vi "ItemByIndex.vi"(7 "LabVIEW Object Type":refnum<class>, 8 "error in (no error)":errorcluster, 10 "Index":i32, 11 "Collection in":refnum<class "CollectionByValue.lvclass">) -> (0 "error out":errorcluster, 1 "found?":bool, 2 "LabVIEW Object":refnum<class>, 3 "Collection out":refnum<class "CollectionByValue.lvclass">)   [LabVIEW 2021, in "Collection.lvlib" / "CollectionByValue.lvclass"]
uses:
  CollectionByValue.lvclass
  CollectionByValue.lvclass/CollectionByValue.ctl
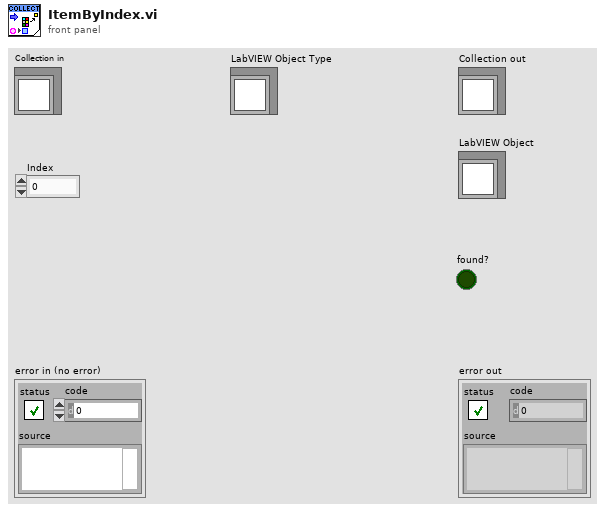
[diagram p1: front panel]
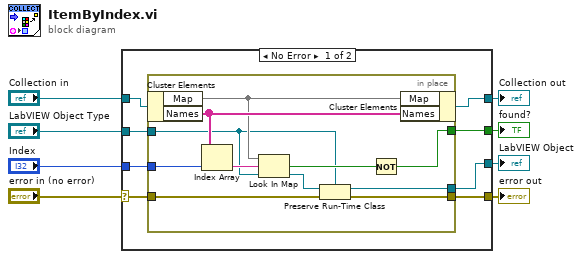
[diagram p0: block diagram]
diagram:
  n1 = case shown="No Error" "error in (no error)" {
    selector: "error in (no error)" -> [w16 w30]
    tunnel: [w15 w30] -> w7
    tunnel: [w13 w29] -> w5
    tunnel: "Collection in" -> [w14 w29]
    tunnel: "LabVIEW Object Type" -> [w12 w28]
    tunnel: [w11 w28] -> w3
    tunnel: "Index" -> [w10 _]
    tunnel: [w9 _] -> w1
    frame No Error {
      n2 = in-place {
        in-place-border: w16 -> [w22]
        in-place-border: [w27] -> w15
        in-place-border: w12 -> [w17]
        in-place-border: [w26] -> w11
        in-place-border: w10 -> [w24]
        in-place-border: [w18] -> w9
        n3 = in-place-cluster #1(w14) -> ("Map"=w20:map{string, refnum<class>}, "Names"=w25:string[])
        n4 = Index Array(array=w25, index=w24) -> (element=w19:string)
        n5 = Look In Map(map=w20, key=w19, default value=w17) -> (key not found?=w23:bool, value=w21:refnum<class>)
        n6 = Preserve Run-Time Class(object in=w21, error in=w22, 2:w17) -> (object out=w26:refnum<class>, error out=w27:errorcluster)
        n7 = Not(x=w23) -> (.not. x?=w18:bool)
        n8 = in-place-cluster #1("Map"=w20, "Names"=w25) -> (w13:refnum<class "CollectionByValue.lvclass">)
      }
    }
    frame Error {
    }
  }
  "error out" <- w7
  "Collection out" <- w5
  "LabVIEW Object" <- w3
  "found?" <- w1
